vi "Driving.vi"(11 "input cluster":T1) -> ()   [LabVIEW 2015]
uses:
  Joystick/ControlsToCommands.ctl
  References/Refnums.vi
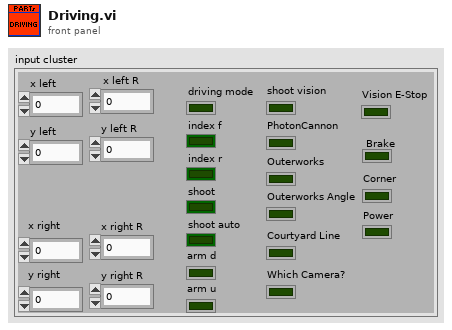
[diagram p1: front panel]
types:
  T1 = typedef "ControlsToCommands.ctl" = cluster{"x left":dbl, "y left":dbl, "x right":dbl, "y right":dbl, "driving mode":bool, "index f":bool, "index r":bool, "shoot":bool, "shoot auto":bool, "arm d":bool, "arm u":bool, "shoot vision":bool, "PhotonCannon":bool, "Outerworks":bool, "Outerworks Angle":bool, "Courtyard Line":bool, "Which Camera?":bool, "Vision E-Stop":bool, "x left R":dbl, "y left R":dbl, "x right R":dbl, "y right R":dbl, "Brake":bool, "Corner":bool, "Power":bool}
  T2 = typedef "WPI_MotorControlDeviceRef.ctl" = cluster{"DeviceStatus":errorcluster, "Type":T3, "PWM":cluster{"PWM Channel":T4, "DeadBand":T5}, "CAN":cluster{"Device Number":u8, "Control Mode":T6, "Semaphore":T7, "Max Vout":dbl, "TalonSRX Control Mode":T8}, "Invert":bool}
  T3 = typedef "WPI_MotorControlType.ctl" = enum16{"PWM", "CAN", "CANTalonSRX"}
  T4 = typedef "FPGA_DIOPWMChannel.ctl" = enum8{"PWM 0", "PWM 1", "PWM 2", "PWM 3", "PWM 4", "PWM 5", "PWM 6", "PWM 7", "PWM 8", "PWM 9", "PWM MXP 0", "PWM MXP 1", "PWM MXP 2", "PWM MXP 3", "PWM MXP 4", "PWM MXP 5", "PWM MXP 6", "PWM MXP 7", "PWM MXP 8", "PWM MXP 9", "Invalid"}
  T5 = typedef "WPI_PWMDeadband.ctl" = cluster{"Name":string, "maxPositivePwm":i32, "minPositivePwm":i32, "centerPwm":i32, "maxNegativePwm":i32, "minNegativePwm":i32, "angularRange":u16}
  T6 = typedef "WPI_CANJaguar_ControlMode.ctl" = enum8{"Percent VBus", "Current", "Speed", "Position", "Voltage"}
  T7 = typedef "Semaphore RefNum" = refnum<k1>
  T8 = typedef "WPI_CANTalonSRX_APIControlMode.ctl" = enum8{"Percent VBus", "Speed", "Position", "Slave", "Unchanged / Invalid", "Voltage Compensation", "Current", "Motion Profile"}
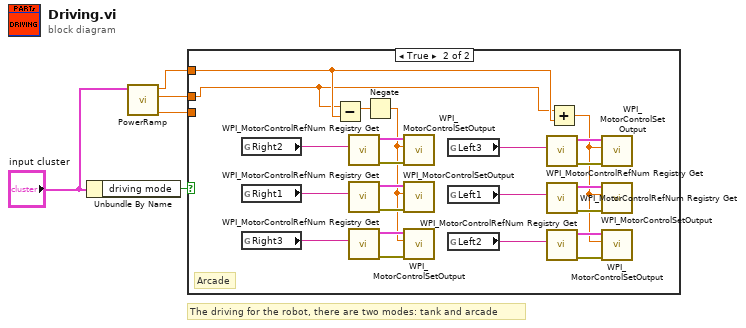
[diagram p0: block diagram]
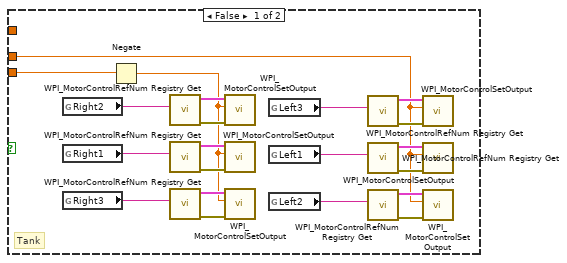
[diagram p2: hidden frame]
diagram:
  # "The driving for the robot, there are two modes: tank and arcade"
  n1 = Unbundle By Name("input cluster") -> ("driving mode"=w5:bool)
  n2 = call "PowerRamp.vi"("input cluster"="input cluster") -> ("y right R"=w1:dbl, "y left R"=w2:dbl, "x left R"=w3:dbl)  [unwired: 7 in, 1 out]
  n3 = case shown="True" w5 {
    tunnel: w3 -> [_ w30]
    tunnel: w2 -> [w8 w29]
    tunnel: w1 -> [w7 _]
    frame False {
      # "Tank"
      n4 = global read "Refnums.vi" "Right2"() -> (w12:string)
      n5 = global read "Refnums.vi" "Right1"() -> (w11:string)
      n6 = global read "Refnums.vi" "Right3"() -> (w17:string)
      n7 = Negate(x=w7) -> (-x=w6:dbl)
      n8 = call <vilib>:"WPI_MotorControlRefNum Registry Get.vi"("refnum name"=w12) -> ("error out"=w14:errorcluster, "MotorControlDevRef"=w13:T2)  [unwired: 9 in]
      n9 = call <vilib>:"WPI_MotorControlRefNum Registry Get.vi"("refnum name"=w11) -> ("error out"=w9:errorcluster, "MotorControlDevRef"=w10:T2)  [unwired: 9 in]
      n10 = call <vilib>:"WPI_MotorControlRefNum Registry Get.vi"("refnum name"=w17) -> ("error out"=w15:errorcluster, "MotorControlDevRef"=w16:T2)  [unwired: 9 in]
      n11 = call <vilib>:"WPI_MotorControlSetOutput.vi"("error in (no error)"=w14, "Output"=w6, "MotorControlDevRef"=w13) -> ()  [unwired: 6 in, 3 out]
      n12 = call <vilib>:"WPI_MotorControlSetOutput.vi"("error in (no error)"=w9, "Output"=w6, "MotorControlDevRef"=w10) -> ()  [unwired: 6 in, 3 out]
      n13 = call <vilib>:"WPI_MotorControlSetOutput.vi"("error in (no error)"=w15, "Output"=w6, "MotorControlDevRef"=w16) -> ()  [unwired: 6 in, 3 out]
      n14 = global read "Refnums.vi" "Left3"() -> (w18:string)
      n15 = global read "Refnums.vi" "Left1"() -> (w24:string)
      n16 = global read "Refnums.vi" "Left2"() -> (w23:string)
      n17 = call <vilib>:"WPI_MotorControlRefNum Registry Get.vi"("refnum name"=w18) -> ("error out"=w20:errorcluster, "MotorControlDevRef"=w19:T2)  [unwired: 9 in]
      n18 = call <vilib>:"WPI_MotorControlRefNum Registry Get.vi"("refnum name"=w24) -> ("error out"=w26:errorcluster, "MotorControlDevRef"=w25:T2)  [unwired: 9 in]
      n19 = call <vilib>:"WPI_MotorControlRefNum Registry Get.vi"("refnum name"=w23) -> ("error out"=w21:errorcluster, "MotorControlDevRef"=w22:T2)  [unwired: 9 in]
      n20 = call <vilib>:"WPI_MotorControlSetOutput.vi"("error in (no error)"=w20, "Output"=w8, "MotorControlDevRef"=w19) -> ()  [unwired: 6 in, 3 out]
      n21 = call <vilib>:"WPI_MotorControlSetOutput.vi"("error in (no error)"=w26, "Output"=w8, "MotorControlDevRef"=w25) -> ()  [unwired: 6 in, 3 out]
      n22 = call <vilib>:"WPI_MotorControlSetOutput.vi"("error in (no error)"=w21, "Output"=w8, "MotorControlDevRef"=w22) -> ()  [unwired: 6 in, 3 out]
    }
    frame True {
      # "Arcade"
      n23 = global read "Refnums.vi" "Right2"() -> (w35:string)
      n24 = global read "Refnums.vi" "Right1"() -> (w34:string)
      n25 = global read "Refnums.vi" "Right3"() -> (w40:string)
      n26 = Subtract(x=w29, y=w30) -> (x-y=w27:dbl)
      n27 = call <vilib>:"WPI_MotorControlRefNum Registry Get.vi"("refnum name"=w35) -> ("error out"=w37:errorcluster, "MotorControlDevRef"=w36:T2)  [unwired: 9 in]
      n28 = call <vilib>:"WPI_MotorControlRefNum Registry Get.vi"("refnum name"=w34) -> ("error out"=w32:errorcluster, "MotorControlDevRef"=w33:T2)  [unwired: 9 in]
      n29 = call <vilib>:"WPI_MotorControlRefNum Registry Get.vi"("refnum name"=w40) -> ("error out"=w38:errorcluster, "MotorControlDevRef"=w39:T2)  [unwired: 9 in]
      n30 = Negate(x=w27) -> (-x=w28:dbl)
      n31 = call <vilib>:"WPI_MotorControlSetOutput.vi"("error in (no error)"=w37, "Output"=w28, "MotorControlDevRef"=w36) -> ()  [unwired: 6 in, 3 out]
      n32 = call <vilib>:"WPI_MotorControlSetOutput.vi"("error in (no error)"=w32, "Output"=w28, "MotorControlDevRef"=w33) -> ()  [unwired: 6 in, 3 out]
      n33 = call <vilib>:"WPI_MotorControlSetOutput.vi"("error in (no error)"=w38, "Output"=w28, "MotorControlDevRef"=w39) -> ()  [unwired: 6 in, 3 out]
      n34 = global read "Refnums.vi" "Left3"() -> (w41:string)
      n35 = global read "Refnums.vi" "Left1"() -> (w47:string)
      n36 = global read "Refnums.vi" "Left2"() -> (w46:string)
      n37 = call <vilib>:"WPI_MotorControlRefNum Registry Get.vi"("refnum name"=w41) -> ("error out"=w43:errorcluster, "MotorControlDevRef"=w42:T2)  [unwired: 9 in]
      n38 = call <vilib>:"WPI_MotorControlRefNum Registry Get.vi"("refnum name"=w47) -> ("error out"=w49:errorcluster, "MotorControlDevRef"=w48:T2)  [unwired: 9 in]
      n39 = call <vilib>:"WPI_MotorControlRefNum Registry Get.vi"("refnum name"=w46) -> ("error out"=w44:errorcluster, "MotorControlDevRef"=w45:T2)  [unwired: 9 in]
      n40 = Add(x=w29, y=w30) -> (x+y=w31:dbl)
      n41 = call <vilib>:"WPI_MotorControlSetOutput.vi"("error in (no error)"=w43, "Output"=w31, "MotorControlDevRef"=w42) -> ()  [unwired: 6 in, 3 out]
      n42 = call <vilib>:"WPI_MotorControlSetOutput.vi"("error in (no error)"=w49, "Output"=w31, "MotorControlDevRef"=w48) -> ()  [unwired: 6 in, 3 out]
      n43 = call <vilib>:"WPI_MotorControlSetOutput.vi"("error in (no error)"=w44, "Output"=w31, "MotorControlDevRef"=w45) -> ()  [unwired: 6 in, 3 out]
    }
  }
